vi "Update Bind RPC Template.vi"(8 "error in (no error)":errorcluster, 11 "Server Library (Library Item) in":refnum<vi>) -> (0 "error out":errorcluster, 3 "Server Library (Library Item) out":refnum<vi>)   [LabVIEW 2019, in "gRPC Scripting Tools.lvlib"]
uses:
  gRPC Scripting Tools.lvlib
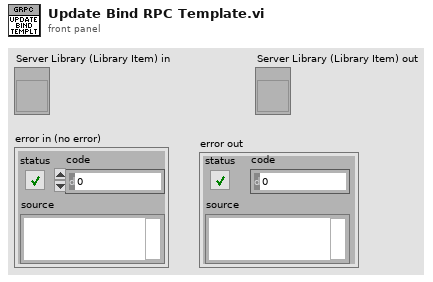
[diagram p1: front panel]
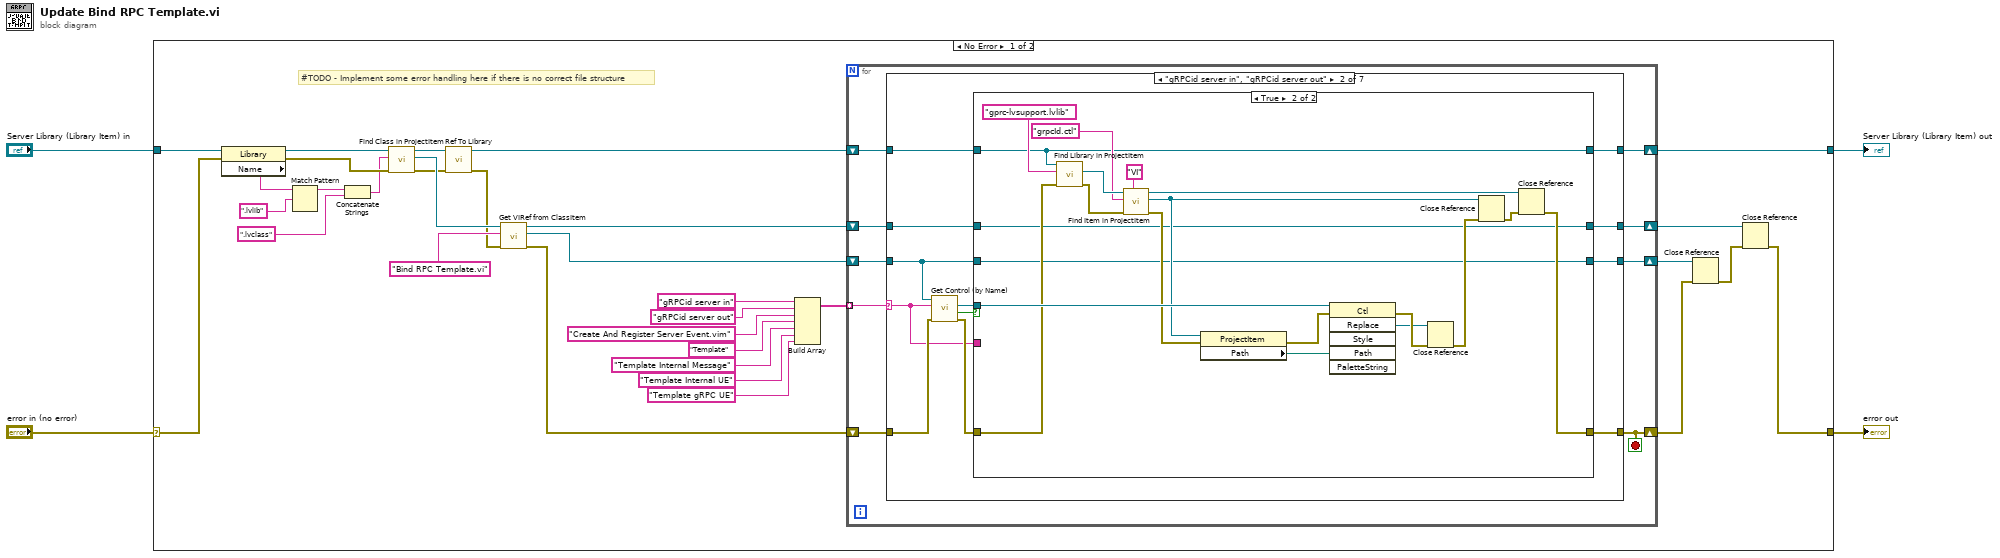
[diagram p0: block diagram]
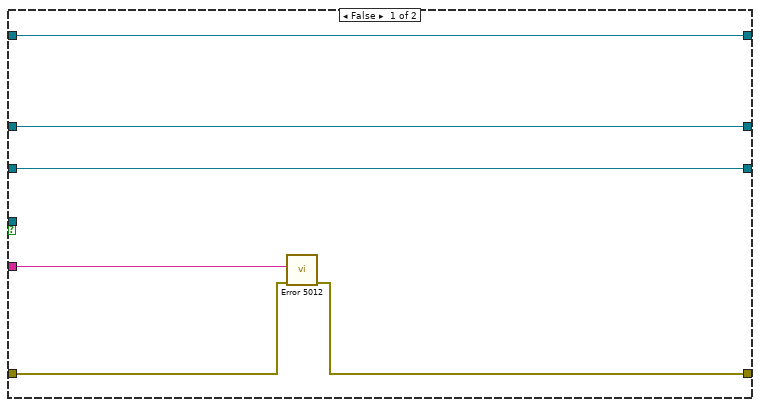
[diagram p3: hidden frame]
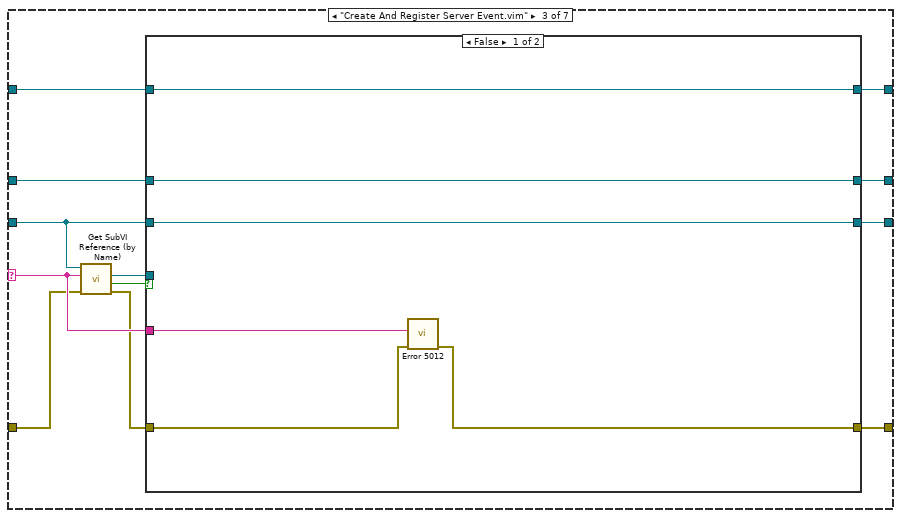
[diagram p4: hidden frame]
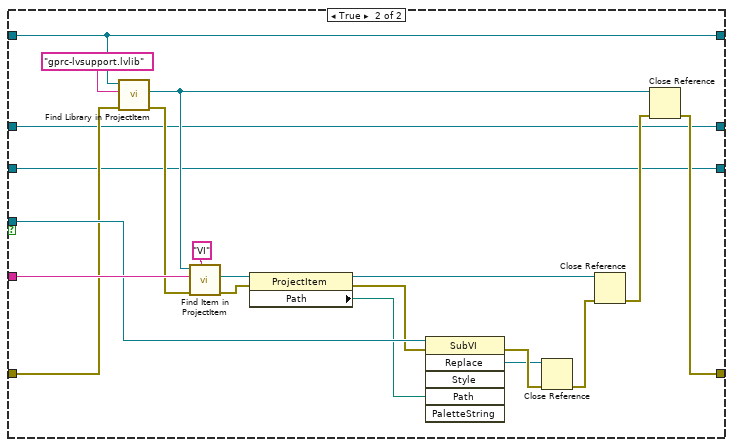
[diagram p5: hidden frame]
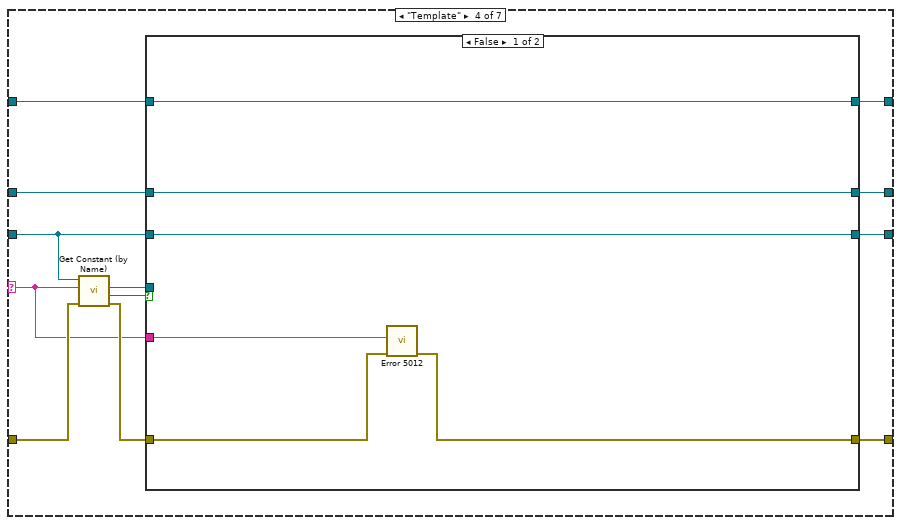
[diagram p6: hidden frame]
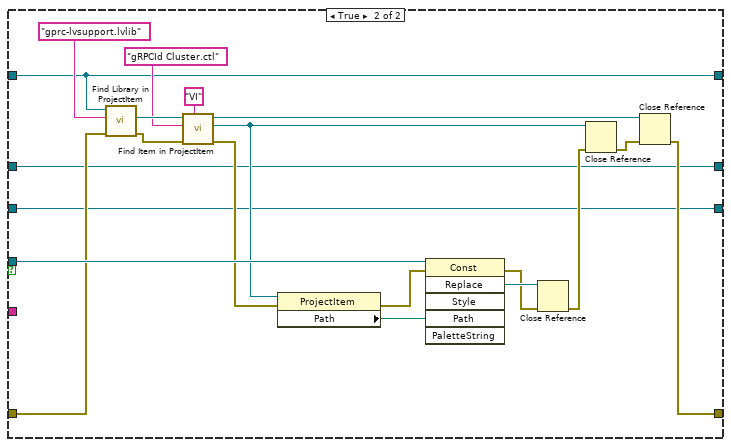
[diagram p7: hidden frame]
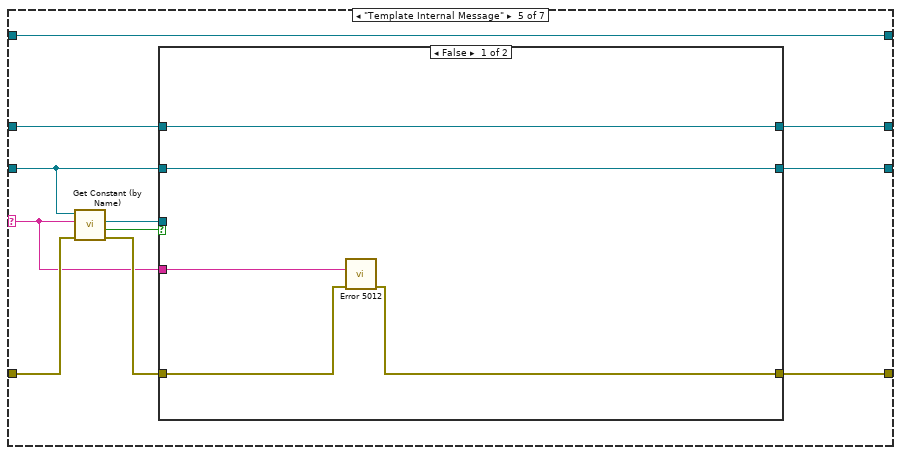
[diagram p8: hidden frame]
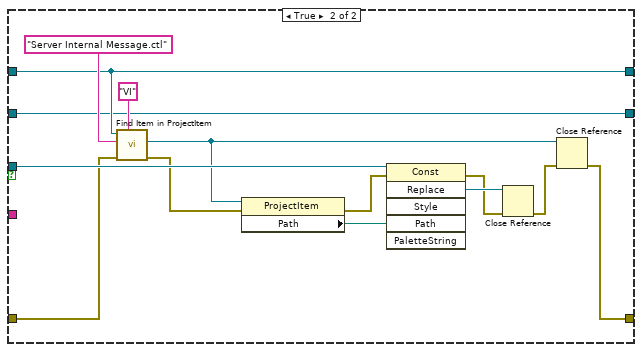
[diagram p9: hidden frame]
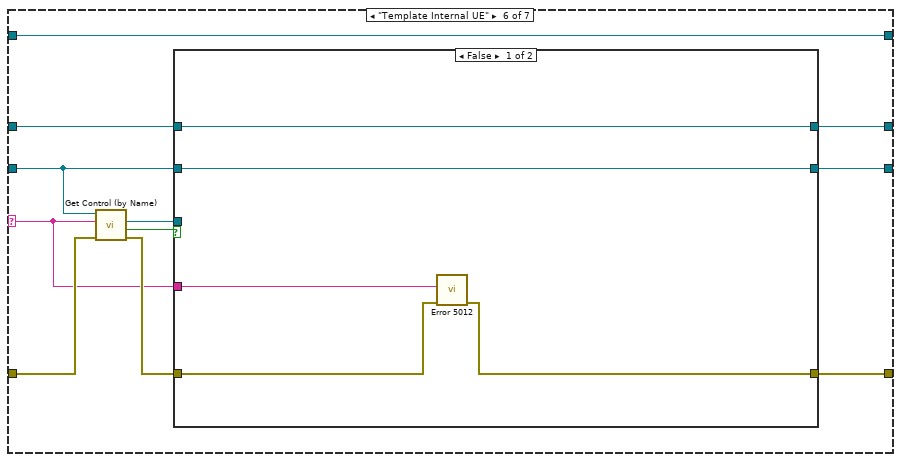
[diagram p10: hidden frame]
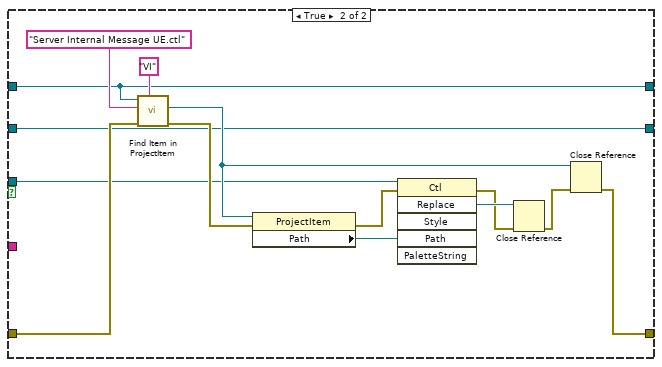
[diagram p11: hidden frame]
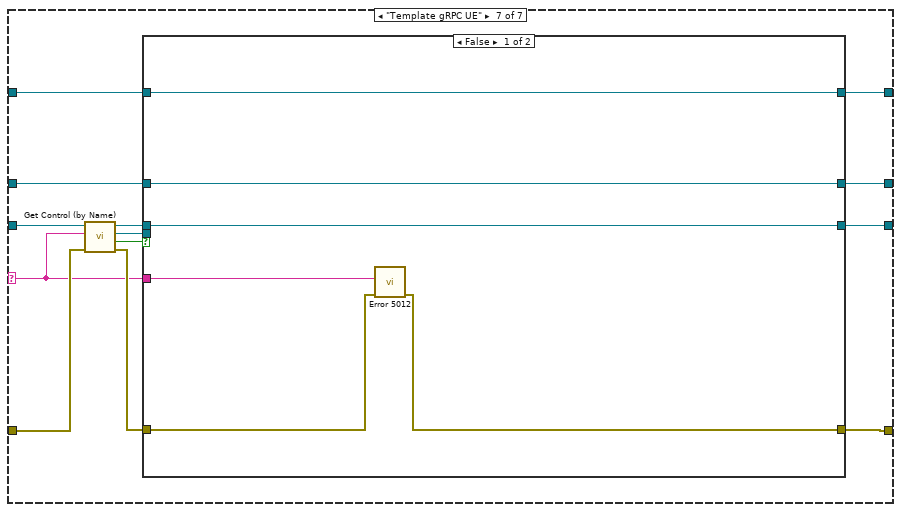
[diagram p12: hidden frame]
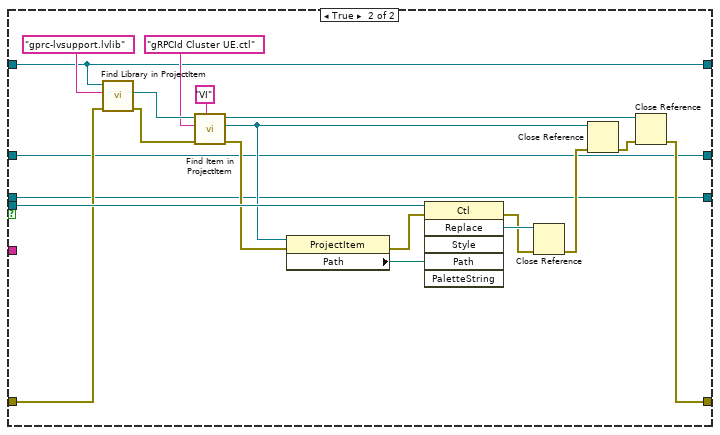
[diagram p13: hidden frame]
diagram:
  n1 = case shown="No Error" "error in (no error)" {
    selector: "error in (no error)" -> [w26 w264]
    tunnel: "Server Library (Library Item) in" -> [w34 w263]
    tunnel: [w8 w264] -> w3
    tunnel: [w10 w263] -> w1
    frame No Error {
      # "#TODO - Implement some error handling here if there is no correct file structure"
      n2 = property class="Library"(reference=w34, error in=w26) -> (reference out=w31:refnum<vi>, error out=w33:errorcluster, "Name"=w27:string)
      n3 = Match Pattern(string=w27, regular expression=".lvlib") -> (before substring=w29:string)  [unwired: 1 in, 3 out]
      n4 = Concatenate Strings(w29, ".lvclass" ("string")) -> (w32:string)
      n5 = call "Find Class in ProjectItem.vi"("error in (no error)"=w33, "Class Name"=w32, "ProjectItem in"=w31) -> ("error out"=w24:errorcluster, "LVClass out"=w36:refnum<vi>, "ProjectItem out"=w25:refnum<vi>)  [unwired: 5 in, 1 out]
      n6 = call "Ref To Library.vi"("error in (no error)"=w24, "ProjectItem in"=w25) -> ("error out"=w23:errorcluster, "Library out"=w15:refnum<vi>)  [unwired: 8 in]
      n7 = call "Get VIRef from ClassItem.vi"("error in (no error)"=w23, "Item Name"="Bind RPC Template.vi", "LVClassLibrary in"=w36) -> ("error out"=w12:errorcluster, "VIref out"=w11:refnum<vi>, "LVClassLibrary out"=w14:refnum<vi>)  [unwired: 5 in, 1 out]
      n8 = Build Array("gRPCid server in" ("Item Name"), "gRPCid server out" ("Item Name"), "Create And Register Server Event.vim" ("Item Name"), "Template" ("Item Name"), "Template Internal Message" ("Item Name"), "Template Internal UE" ("Item Name"), "Template gRPC UE" ("Item Name")) -> (w13:string[])
      n9 = for {
        shift-right: [w43] -> w10
        shift-left: w15 -> [w44]
        tunnel: w13 -> [w45] mode=indexing
        shift-right: [w37] -> w6
        shift-left: w12 -> [w42]
        shift-right: [w39] -> w9
        shift-left: w14 -> [w40]
        shift-right: [w38] -> w7
        shift-left: w11 -> [w41]
        stop <- w37 stop-if-true
        n10 = case shown="\"gRPCid server in\", \"gRPCid server out\"" w45 {
          selector: w45 -> [_ w50 w98 w126 w164 w194 w224]
          tunnel: w44 -> [w49 w61 w99 w137 w174 w204 w233]
          tunnel: [w49 w51 w88 w127 w174 w204 w229] -> w43
          tunnel: w41 -> [w46 w55 w92 w131 w166 w197 w236]
          tunnel: w42 -> [w48 w59 w96 w135 w172 w202 w235]
          tunnel: [w48 w57 w94 w133 w171 w203 w231] -> w37
          tunnel: w40 -> [w47 w53 w90 w129 w169 w199 w228]
          tunnel: [w47 w52 w89 w128 w167 w195 w227] -> w39
          tunnel: [w46 w54 w91 w130 w165 w196 w225] -> w38
          frame "None", Default {
          }
          frame "gRPCid server in", "gRPCid server out" {
            n11 = call "Get Control (by Name).vi"("error in (no error)"=w59, "Control Label"=w50, "Owner VI in"=w55) -> ("error out"=w58:errorcluster, "Found ?"=w56:bool, "Control Refnum"=w60:refnum<vi>)  [unwired: 5 in, 1 out]
            n12 = case shown="True" w56 {
              tunnel: w61 -> [w67 w68]
              tunnel: w60 -> [_ w83]
              tunnel: w58 -> [w64 w81]
              tunnel: [w62 w71] -> w57
              tunnel: w55 -> [w65 w70]
              tunnel: [w65 w70] -> w54
              tunnel: w53 -> [w66 w69]
              tunnel: [w66 w69] -> w52
              tunnel: [w67 w68] -> w51
              tunnel: w50 -> [w63 _]
              frame False {
                n13 = call "Error 5012.vi"("error in (no error)"=w64, "Element Name"=w63) -> ("error out"=w62:errorcluster)  [unwired: 9 in]
              }
              frame True {
                n14 = call "Find Library in ProjectItem.vi"("error in (no error)"=w81, "Library Name"="gprc-lvsupport.lvlib", "ProjectItem in"=w68) -> ("error out"=w80:errorcluster, "Library out"=w86:refnum<vi>)  [unwired: 5 in, 2 out]
                n15 = call "Find Item in ProjectItem.vi"("Item Type"="VI", "error in (no error)"=w80, "Name"="grpcId.ctl", "ProjectItem in"=w86) -> ("error out"=w79:errorcluster, "Item Refnum out"=w74:refnum<vi>, "ProjectItem out"=w72:refnum<vi>)  [unwired: 4 in, 1 out]
                n16 = property class="ProjectItem"(reference=w74, error in=w79) -> (error out=w76:errorcluster, "Path"=w82:path)  [unwired: 1 out]
                n17 = invoke class="Ctl" method="Replace"(reference=w83, error in=w76, "Path"=w82) -> (error out=w78:errorcluster, "Replace"=w77:refnum<vi>)  [unwired: 3 in, 4 out]
                n18 = Close Reference(reference=w77, error in (no error)=w78) -> (error out=w75:errorcluster)
                n19 = Close Reference(reference=w74, error in (no error)=w75) -> (error out=w73:errorcluster)
                n20 = Close Reference(reference=w72, error in (no error)=w73) -> (error out=w71:errorcluster)
              }
            }
          }
          frame "Create And Register Server Event.vim" {
            n21 = call "Get SubVI Reference (by Name).vi"("error in (no error)"=w96, "SubVI Name"=w98, "Owner VI in"=w92) -> ("error out"=w95:errorcluster, "Found ?"=w93:bool, "SubVI Refnum out"=w97:refnum<vi>)  [unwired: 5 in, 1 out]
            n22 = case shown="False" w93 {
              tunnel: w99 -> [w105 w106]
              tunnel: w98 -> [w101 w123]
              tunnel: w97 -> [_ w122]
              tunnel: w95 -> [w102 w117]
              tunnel: [w100 w109] -> w94
              tunnel: w92 -> [w103 w108]
              tunnel: [w103 w108] -> w91
              tunnel: w90 -> [w104 w107]
              tunnel: [w104 w107] -> w89
              tunnel: [w105 w106] -> w88
              frame False {
                n23 = call "Error 5012.vi"("error in (no error)"=w102, "Element Name"=w101) -> ("error out"=w100:errorcluster)  [unwired: 9 in]
              }
              frame True {
                n24 = call "Find Library in ProjectItem.vi"("error in (no error)"=w117, "Library Name"="gprc-lvsupport.lvlib", "ProjectItem in"=w106) -> ("error out"=w116:errorcluster, "Library out"=w111:refnum<vi>)  [unwired: 5 in, 2 out]
                n25 = call "Find Item in ProjectItem.vi"("Item Type"="VI", "error in (no error)"=w116, "Name"=w123, "ProjectItem in"=w111) -> ("error out"=w115:errorcluster, "Item Refnum out"=w121:refnum<vi>)  [unwired: 4 in, 2 out]
                n26 = property class="ProjectItem"(reference=w121, error in=w115) -> (reference out=w113:refnum<vi>, error out=w114:errorcluster, "Path"=w120:path)
                n27 = invoke class="SubVI" method="Replace"(reference=w122, error in=w114, "Path"=w120) -> (error out=w119:errorcluster, "Replace"=w118:refnum<vi>)  [unwired: 3 in, 4 out]
                n28 = Close Reference(reference=w118, error in (no error)=w119) -> (error out=w112:errorcluster)
                n29 = Close Reference(reference=w113, error in (no error)=w112) -> (error out=w110:errorcluster)
                n30 = Close Reference(reference=w111, error in (no error)=w110) -> (error out=w109:errorcluster)
              }
            }
          }
          frame "Template" {
            n31 = call "Get Constant (by Name).vi"("error in (no error)"=w135, "Constant Label"=w126, "Owner VI in"=w131) -> ("error out"=w134:errorcluster, "Found ?"=w132:bool, "Const ref out"=w136:refnum<vi>)  [unwired: 5 in, 1 out]
            n32 = case shown="False" w132 {
              tunnel: w137 -> [w143 w144]
              tunnel: w136 -> [_ w157]
              tunnel: w134 -> [w139 w150]
              tunnel: [w138 w147] -> w133
              tunnel: w131 -> [w141 w146]
              tunnel: [w141 w146] -> w130
              tunnel: w129 -> [w142 w145]
              tunnel: [w142 w145] -> w128
              tunnel: [w143 w144] -> w127
              tunnel: w126 -> [w140 _]
              frame False {
                n33 = call "Error 5012.vi"("error in (no error)"=w139, "Element Name"=w140) -> ("error out"=w138:errorcluster)  [unwired: 9 in]
              }
              frame True {
                n34 = call "Find Library in ProjectItem.vi"("error in (no error)"=w150, "Library Name"="gprc-lvsupport.lvlib", "ProjectItem in"=w144) -> ("error out"=w149:errorcluster, "Library out"=w162:refnum<vi>)  [unwired: 5 in, 2 out]
                n35 = call "Find Item in ProjectItem.vi"("Item Type"="VI", "error in (no error)"=w149, "Name"="gRPCId Cluster.ctl", "ProjectItem in"=w162) -> ("error out"=w148:errorcluster, "Item Refnum out"=w154:refnum<vi>, "ProjectItem out"=w152:refnum<vi>)  [unwired: 4 in, 1 out]
                n36 = property class="ProjectItem"(reference=w154, error in=w148) -> (error out=w158:errorcluster, "Path"=w159:path)  [unwired: 1 out]
                n37 = invoke class="Const" method="Replace"(reference=w157, error in=w158, "Path"=w159) -> (error out=w155:errorcluster, "Replace"=w156:refnum<vi>)  [unwired: 3 in, 4 out]
                n38 = Close Reference(reference=w156, error in (no error)=w155) -> (error out=w153:errorcluster)
                n39 = Close Reference(reference=w154, error in (no error)=w153) -> (error out=w151:errorcluster)
                n40 = Close Reference(reference=w152, error in (no error)=w151) -> (error out=w147:errorcluster)
              }
            }
          }
          frame "Template Internal Message" {
            n41 = call "Get Constant (by Name).vi"("error in (no error)"=w172, "Constant Label"=w164, "Owner VI in"=w166) -> ("error out"=w170:errorcluster, "Found ?"=w168:bool, "Const ref out"=w173:refnum<vi>)  [unwired: 5 in, 1 out]
            n42 = case shown="False" w168 {
              tunnel: w173 -> [_ w189]
              tunnel: [w175 w183] -> w171
              tunnel: w170 -> [w176 w182]
              tunnel: w169 -> [w179 w181]
              tunnel: [w179 w181] -> w167
              tunnel: w166 -> [w178 w180]
              tunnel: [w178 w180] -> w165
              tunnel: w164 -> [w177 _]
              frame False {
                n43 = call "Error 5012.vi"("error in (no error)"=w176, "Element Name"=w177) -> ("error out"=w175:errorcluster)  [unwired: 9 in]
              }
              frame True {
                n44 = call "Find Item in ProjectItem.vi"("Item Type"="VI", "error in (no error)"=w182, "Name"="Server Internal Message.ctl", "ProjectItem in"=w181) -> ("error out"=w184:errorcluster, "Item Refnum out"=w186:refnum<vi>)  [unwired: 4 in, 2 out]
                n45 = property class="ProjectItem"(reference=w186, error in=w184) -> (error out=w190:errorcluster, "Path"=w191:path)  [unwired: 1 out]
                n46 = invoke class="Const" method="Replace"(reference=w189, error in=w190, "Path"=w191) -> (error out=w187:errorcluster, "Replace"=w188:refnum<vi>)  [unwired: 3 in, 4 out]
                n47 = Close Reference(reference=w188, error in (no error)=w187) -> (error out=w185:errorcluster)
                n48 = Close Reference(reference=w186, error in (no error)=w185) -> (error out=w183:errorcluster)
              }
            }
          }
          frame "Template Internal UE" {
            n49 = call "Get Control (by Name).vi"("error in (no error)"=w202, "Control Label"=w194, "Owner VI in"=w197) -> ("error out"=w201:errorcluster, "Found ?"=w198:bool, "Control Refnum"=w200:refnum<vi>)  [unwired: 5 in, 1 out]
            n50 = case shown="False" w198 {
              tunnel: [w206 w214] -> w203
              tunnel: w201 -> [w207 w213]
              tunnel: w200 -> [_ w212]
              tunnel: w199 -> [w209 w210]
              tunnel: w197 -> [w208 w211]
              tunnel: [w208 w211] -> w196
              tunnel: [w209 w210] -> w195
              tunnel: w194 -> [w205 _]
              frame False {
                n51 = call "Error 5012.vi"("error in (no error)"=w207, "Element Name"=w205) -> ("error out"=w206:errorcluster)  [unwired: 9 in]
              }
              frame True {
                n52 = call "Find Item in ProjectItem.vi"("Item Type"="VI", "error in (no error)"=w213, "Name"="Server Internal Message UE.ctl", "ProjectItem in"=w210) -> ("error out"=w215:errorcluster, "Item Refnum out"=w217:refnum<vi>)  [unwired: 4 in, 2 out]
                n53 = property class="ProjectItem"(reference=w217, error in=w215) -> (error out=w220:errorcluster, "Path"=w221:path)  [unwired: 1 out]
                n54 = invoke class="Ctl" method="Replace"(reference=w212, error in=w220, "Path"=w221) -> (error out=w218:errorcluster, "Replace"=w219:refnum<vi>)  [unwired: 3 in, 4 out]
                n55 = Close Reference(reference=w219, error in (no error)=w218) -> (error out=w216:errorcluster)
                n56 = Close Reference(reference=w217, error in (no error)=w216) -> (error out=w214:errorcluster)
              }
            }
          }
          frame "Template gRPC UE" {
            n57 = call "Get Control (by Name).vi"("error in (no error)"=w235, "Control Label"=w224, "Owner VI in"=w236) -> ("error out"=w232:errorcluster, "Found ?"=w230:bool, "Control Refnum"=w234:refnum<vi>, "Owner VI out"=w226:refnum<vi>)  [unwired: 5 in]
            n58 = case shown="False" w230 {
              tunnel: w234 -> [_ w257]
              tunnel: w233 -> [w242 w245]
              tunnel: w232 -> [w239 w251]
              tunnel: [w237 w246] -> w231
              tunnel: [w242 w245] -> w229
              tunnel: w228 -> [w241 w244]
              tunnel: [w241 w244] -> w227
              tunnel: w226 -> [w240 w243]
              tunnel: [w240 w243] -> w225
              tunnel: w224 -> [w238 _]
              frame False {
                n59 = call "Error 5012.vi"("error in (no error)"=w239, "Element Name"=w238) -> ("error out"=w237:errorcluster)  [unwired: 9 in]
              }
              frame True {
                n60 = call "Find Library in ProjectItem.vi"("error in (no error)"=w251, "Library Name"="gprc-lvsupport.lvlib", "ProjectItem in"=w245) -> ("error out"=w252:errorcluster, "Library out"=w255:refnum<vi>)  [unwired: 5 in, 2 out]
                n61 = call "Find Item in ProjectItem.vi"("Item Type"="VI", "error in (no error)"=w252, "Name"="gRPCId Cluster UE.ctl", "ProjectItem in"=w255) -> ("error out"=w250:errorcluster, "Item Refnum out"=w249:refnum<vi>, "ProjectItem out"=w248:refnum<vi>)  [unwired: 4 in, 1 out]
                n62 = property class="ProjectItem"(reference=w249, error in=w250) -> (error out=w261:errorcluster, "Path"=w262:path)  [unwired: 1 out]
                n63 = invoke class="Ctl" method="Replace"(reference=w257, error in=w261, "Path"=w262) -> (error out=w259:errorcluster, "Replace"=w260:refnum<vi>)  [unwired: 3 in, 4 out]
                n64 = Close Reference(reference=w260, error in (no error)=w259) -> (error out=w258:errorcluster)
                n65 = Close Reference(reference=w249, error in (no error)=w258) -> (error out=w247:errorcluster)
                n66 = Close Reference(reference=w248, error in (no error)=w247) -> (error out=w246:errorcluster)
              }
            }
          }
        }
      }
      n67 = Close Reference(reference=w7, error in (no error)=w6) -> (error out=w5:errorcluster)
      n68 = Close Reference(reference=w9, error in (no error)=w5) -> (error out=w8:errorcluster)
    }
    frame Error {
    }
  }
  "error out" <- w3
  "Server Library (Library Item) out" <- w1
